vi "Player Info.vi"(11 "Line Dancer in":refnum<class "Fractal.lvclass">) -> (1 "Victory Speech":string, 2 "Name":string, 3 "Line Dancer out":refnum<class "Fractal.lvclass">)   [LabVIEW 2015, in "Fractal.lvclass"]
uses:
  Fractal.lvclass
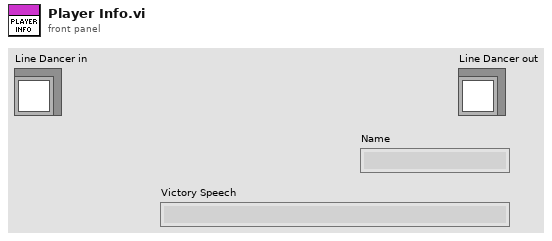
[diagram p1: front panel]
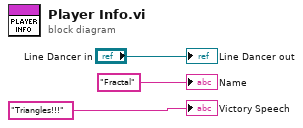
[diagram p0: block diagram]
diagram:
  "Line Dancer out" <- "Line Dancer in"
  "Name" <- "Fractal" ("Name")
  "Victory Speech" <- "Triangles!!!" ("Victory Speech")
